vi "_CSMObj-Update ChainData.vi"(8 "Error In":errorcluster caption="error in (no error)", 11 "CSMObj In":T1) -> (0 "error out":errorcluster, 3 "CSMObj Out":T1)   [LabVIEW 2017, in "Communicable State Machine.lvlib"]
uses:
  Communicable State Machine.lvlib
  _CSMObj.ctl
  _CSMObj-Info.ctl
  Typedef/_CSM_MODE.ctl
  _CSMObj-Refs.ctl
  _CSMObj-Data.ctl
  Priority Queue/Priority Queue.ctl
  Typedef/_Cross CSM State Data.ctl
  Typedef/_CSM_MSG_TYPE.ctl
  Typedef/_Cross CSM State Response.ctl
  Typedef/_CSM_Response Source Message.ctl
  Priority Queue/def-Data(LowPRI-Q).ctl
  _CSMObj-ModeData.ctl
  Typedef/_CSM Status Change Event Data.ctl
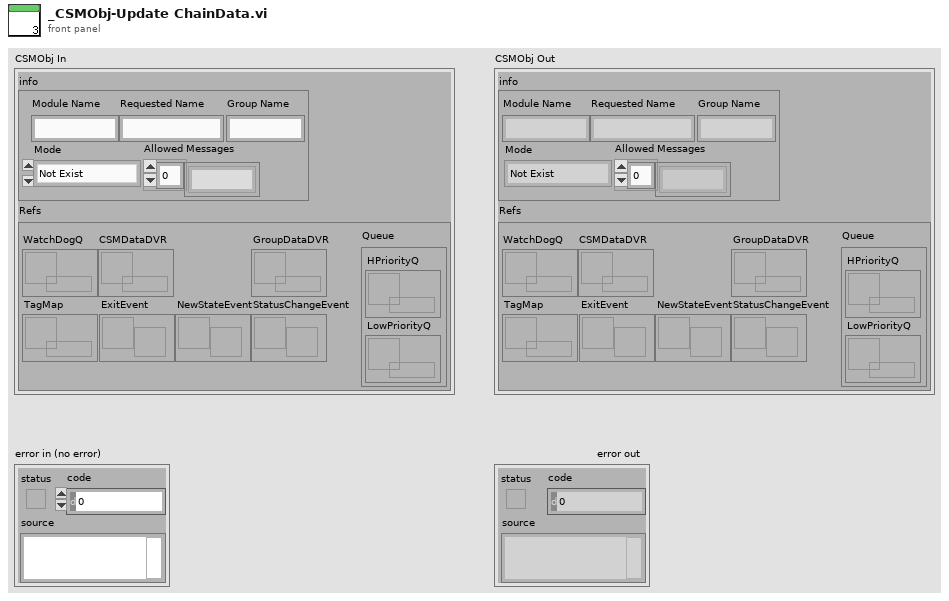
[diagram p1: front panel]
types:
  T1 = typedef "Communicable State Machine.lvlib/_CSMObj.ctl" = cluster{"info":T2, "Refs":T4}
  T2 = typedef "Communicable State Machine.lvlib/_CSMObj-Info.ctl" = cluster{"Module Name":string, "Requested Name":string, "Group Name":string, "Mode":T3, "Allowed Messages":string[]}
  T3 = typedef "Communicable State Machine.lvlib/_CSM_MODE.ctl" = enum16{"Not Exist", "Stand Alone", "CSM", "Worker", "Worker Agent", "Chain Node", "Chain"}
  T4 = typedef "Communicable State Machine.lvlib/_CSMObj-Refs.ctl" = cluster{"WatchDogQ":refnum<queue>, "CSMDataDVR":refnum<data-value>, "Queue":T5, "GroupDataDVR":refnum<data-value>, "TagMap":refnum<data-value>, "ExitEvent":refnum<user-event>, "NewStateEvent":refnum<user-event>, "StatusChangeEvent":refnum<user-event>}
  T5 = typedef "Communicable State Machine.lvlib/Priority Queue.ctl" = cluster{"HPriorityQ":refnum<queue>, "LowPriorityQ":refnum<queue>}
  T6 = cluster{"Module Name":string, "Allowed Messages":string[]}
  T7 = typedef "Communicable State Machine.lvlib/_CSMObj-ModeData.ctl" = cluster{"CSMDataDVR":refnum<data-value>[], "Messages of Chain Nodes":cluster{"Module Name":string, "Allowed Messages":string[]}[], "Chain Message Mapping Map":variant}
  T8 = cluster{"Module Name":string, "Allowed Messages":string[]}[]
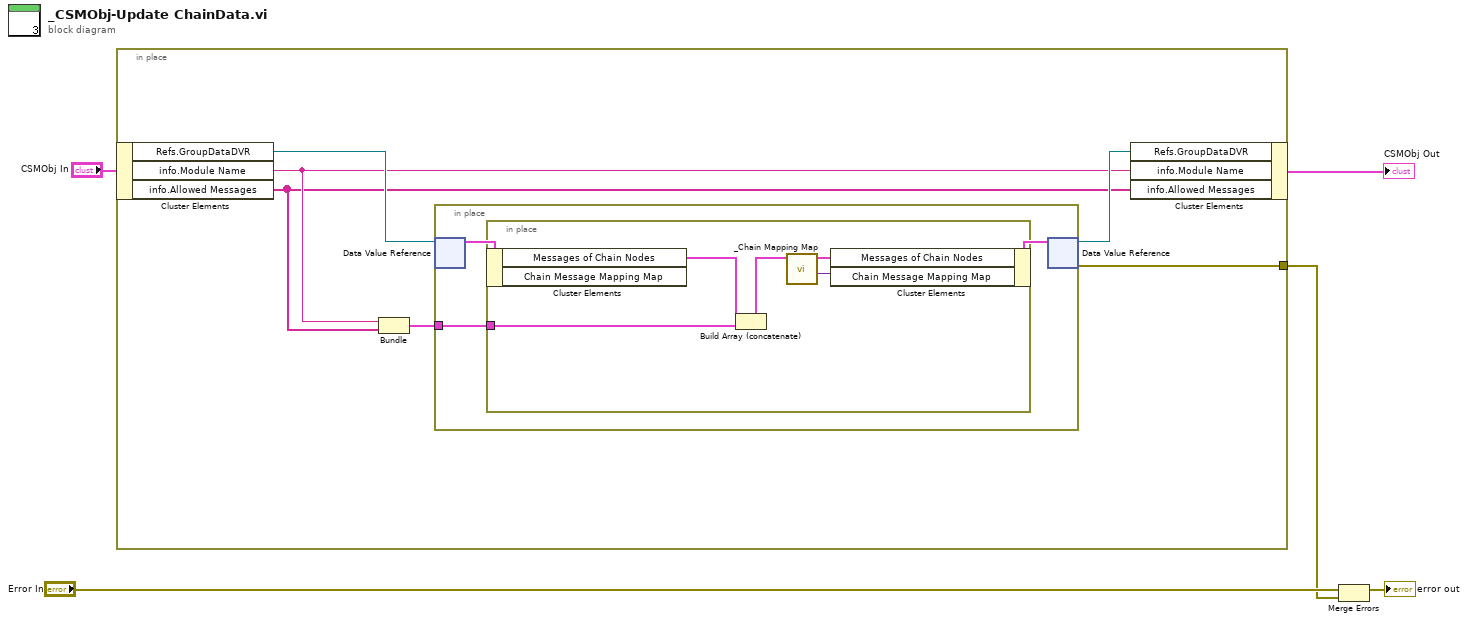
[diagram p0: block diagram]
diagram:
  n1 = in-place "In Place Element Structure" {
    in-place-border: [w6] -> w1
    n2 = in-place-cluster #1("CSMObj In") -> ("Refs.GroupDataDVR"=w11:refnum<data-value>, "info.Module Name"=w9:string, "info.Allowed Messages"=w8:string[])
    n3 = Bundle("Module Name"=w9, "Allowed Messages"=w8) -> (w7:T6)  [unwired: 1 in]
    n4 = in-place {
      in-place-border: w7 -> [w12]
      n5 = in-place-dvr #2(w11) -> (w14:T7)  [unwired: 1 out]
      n6 = in-place {
        in-place-border: w12 -> [w15]
        n7 = in-place-cluster #3(w14) -> ("Messages of Chain Nodes"=w19:T8)  [unwired: 1 out]
        n8 = Build Array (concatenate)(w19, w15) -> (w18:T8)
        n9 = call "_Chain Mapping Map.vi"("Messages of Chain Nodes"=w18) -> ("Variant"=w16:variant, "Messages of Chain Nodes (Dup)"=w17:T8)  [unwired: 9 in]
        n10 = in-place-cluster #3("Messages of Chain Nodes"=w17, "Chain Message Mapping Map"=w16) -> (w13:T7)
      }
      n11 = in-place-dvr #2(w13) -> (w10:refnum<data-value>, w6:errorcluster)
    }
    n12 = in-place-cluster #1("Refs.GroupDataDVR"=w10, "info.Module Name"=w9, "info.Allowed Messages"=w8) -> (→"CSMObj Out":T1)
  }
  n13 = Merge Errors("Error In", w1) -> (→"error out":errorcluster)
